vi "USB3 Initialize Library.vi"(7 "error in (no error)":errorcluster) -> (0 "error out":errorcluster, 3 "function return":i32)   [LabVIEW 2013, in "Octoplus_LIDAR.lvlib"]
doc: "CAMCMOSOCTUSB3_API int __cdecl USB3_InitializeLibrary(void);"
uses:
  <userlib>/Octoplus_LIDAR/Octoplus_LIDAR.lvlib
  <userlib>/Octoplus_LIDAR/CamCmosOctUsb3.dll
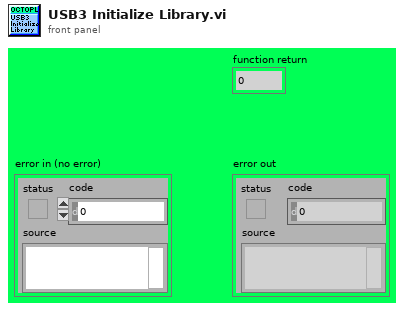
[diagram p1: front panel]
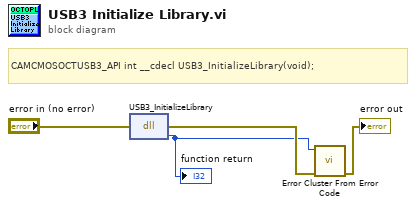
[diagram p0: block diagram]
diagram:
  # "CAMCMOSOCTUSB3_API int __cdecl USB3_InitializeLibrary(void);"
  n1 = dll-call lib="C:/Program Files/National Instruments/LabVIEW 2013/user.lib/Octoplus_LIDAR/CamCmosOctUsb3.*" fn="USB3_InitializeLibrary"(error in="error in (no error)") -> (error out=w3:errorcluster, w1:i32)  [unwired: 2 in, 1 out]
  "function return" <- w1
  n2 = call <vilib>:"Error Cluster From Error Code.vi"("error in (no error)"=w3, "error code (0)"=w1) -> ("error out"=→"error out":errorcluster)  [unwired: 7 in]
